vi "运行环境动态添加删除游标（游标图例）.vi"() -> ()   [LabVIEW 2012]
uses:
  <vilib>/Utility/miscctls.llb/LVCursorListTypeDef.ctl
  <vilib>/measure/NI_MABase.lvlib
panel:
  out "游标列表":T1
  in  "停止":bool
  out "波形图":waveform(dbl)(graph)
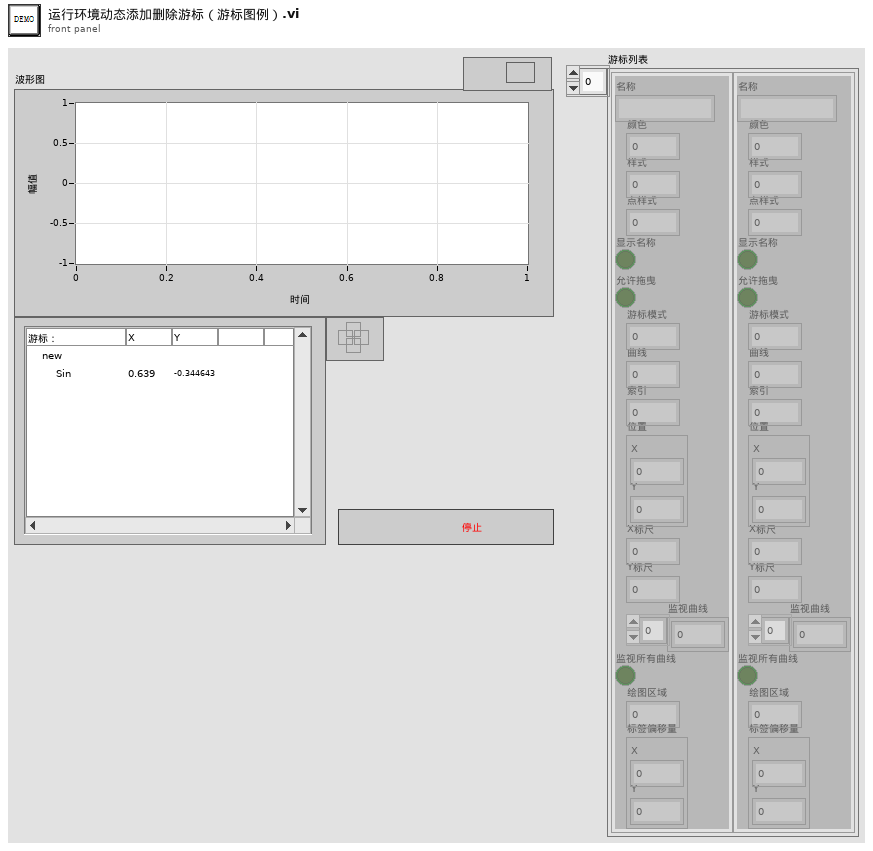
[diagram p1: front panel]
types:
  T1 = typedef "LVCursorListTypeDef.ctl" = cluster{"Name":string, "Color":u32, "Style":u8, "Point Style":u8, "Name Visible":bool, "Allow Drag":bool, "Cursor Mode":u32, "Plot":i32, "Index":i32, "Position":cluster{"X":dbl, "Y":dbl}, "X Scale":u32, "Y Scale":u32, "Watch Plots":i32[], "Watch All Plots":bool, "Plot Area":i32, "Label Offset":cluster{"X":dbl, "Y":dbl}}[]
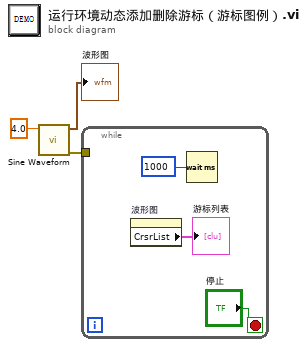
[diagram p0: block diagram]
diagram:
  n1 = call <vilib>:"Sine Waveform.vi"("frequency"=4.0) -> ("error out"=w1:errorcluster, "signal out"=→"波形图":waveform(dbl))  [unwired: 9 in]
  n2 = while {
    tunnel: w1 -> [_]
    stop <- "停止" stop-if-true
    n3 = property on="波形图" class="WFGraph (严格)"() -> ("CrsrList"=→"游标列表":T1)  [unwired: 2 in, 2 out]
    n4 = Wait (ms)(milliseconds to wait=u32 1000 ("等待时间（毫秒）")) -> ()  [unwired: 1 out]
  }
